vi "WSVCAP SHL Host LL I2C Convert 4 Bytes to Status and Capacitance.vi"(0 "C:1-24 Read Data [U8]":u8[][](array[numeric]) format="%.0x") -> (4 "AD7747 Values":string[][](table))   [LabVIEW 2017]
panel:
  out "Data Headers":u8[](array[numeric])=[1, 2, 3, 4, 5, 6, 7, 8, 9, 10, 11, 12, 12, 14, 15, 16, 17, 18, 19, 20, 21, 22, 23, 24, 25, 26, 27, 28, 29, 30, 31, 32, 33, 34, 35, 36]
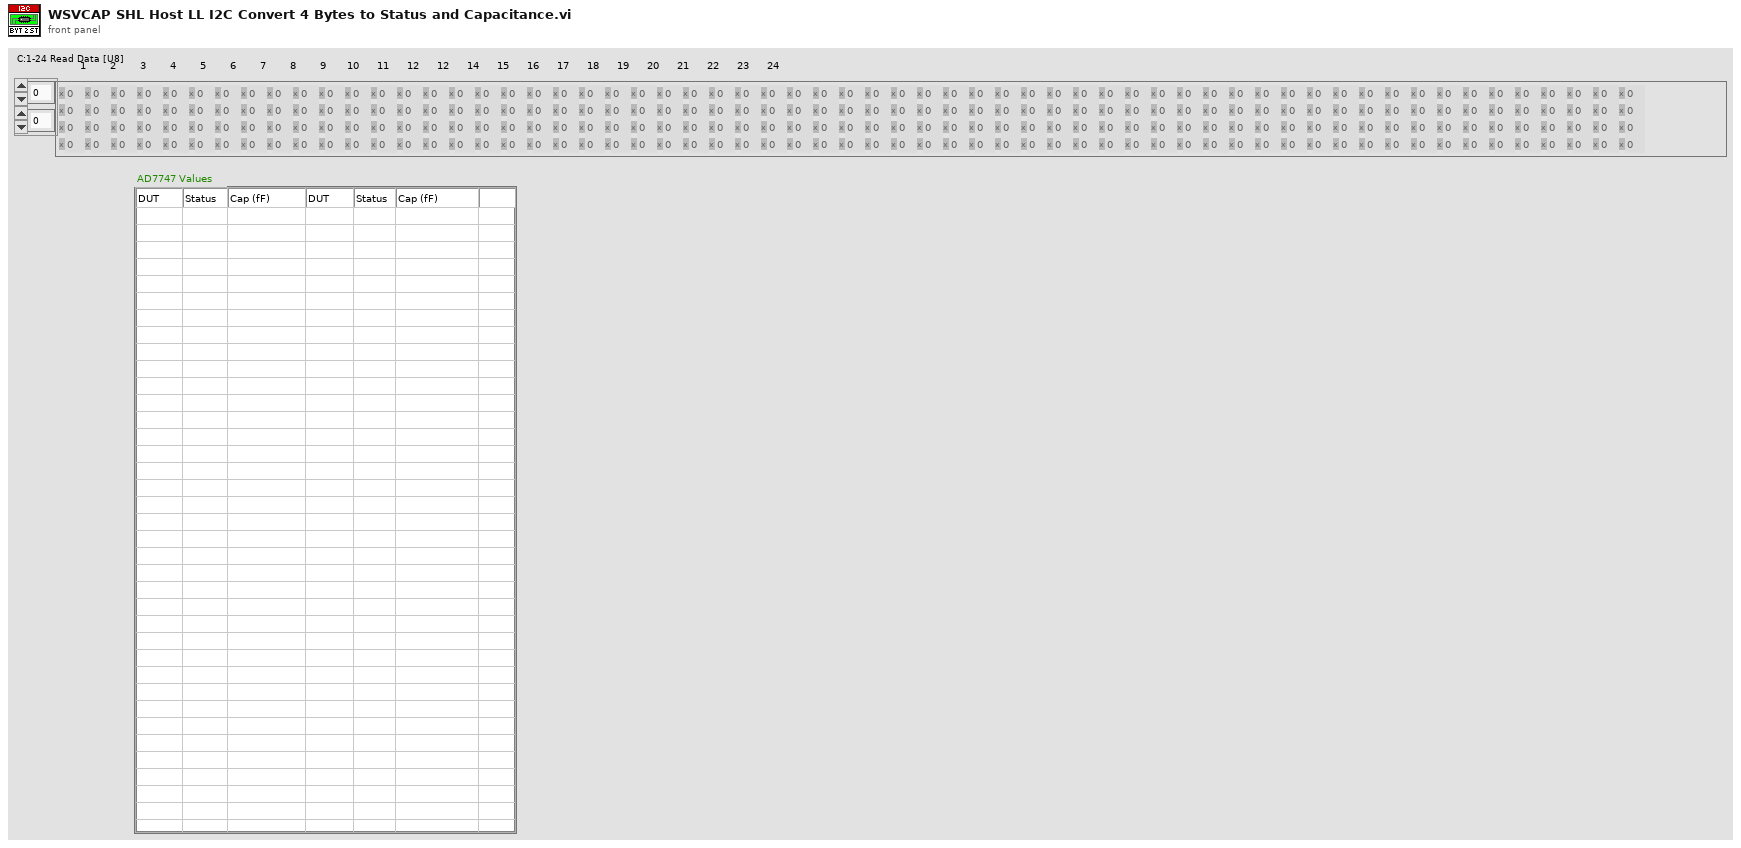
[diagram p1: front panel]
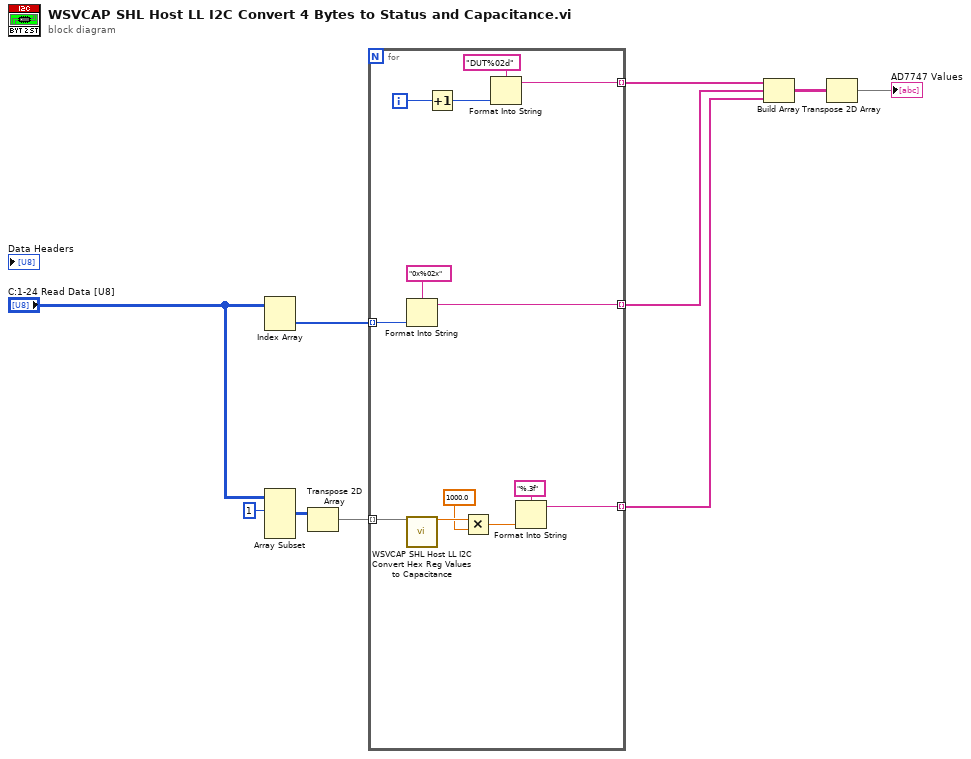
[diagram p0: block diagram]
diagram:
  n1 = Index Array(array="C:1-24 Read Data [U8]") -> (element=w10:u8[])  [unwired: 2 in]
  n2 = Array Subset(array="C:1-24 Read Data [U8]", index (row)=1 ("index")) -> (w8:u8[][])  [unwired: 3 in]
  n3 = Transpose 2D Array(2D array=w8) -> (transposed array=w7:u8[][])
  n4 = for {
    tunnel: w10 -> [w22] mode=indexing
    tunnel: w7 -> [w23] mode=indexing
    tunnel: [w21] -> w3 mode=indexing
    tunnel: [w20] -> w4 mode=indexing
    tunnel: [w15] -> w1 mode=indexing
    i -> [w16]
    n5 = Format Into String(format string="0x%02x", w22) -> (resulting string=w21:string)  [unwired: 2 in, 1 out]
    n6 = call "WSVCAP SHL Host LL I2C Convert Hex Reg Values to Capacitance.vi"("Bytes (H-M-L)"=w23) -> ("Capacitance (pF)"=w13:dbl)  [unwired: 14 in]
    n7 = Increment(x=w16) -> (x+1=w17:i32)
    n8 = Multiply(x=w13, y=1000.0) -> (x*y=w11:dbl)
    n9 = Format Into String(format string="DUT%02d", w17) -> (resulting string=w15:string)  [unwired: 2 in, 1 out]
    n10 = Format Into String(format string="%.3f", w11) -> (resulting string=w20:string)  [unwired: 2 in, 1 out]
  }
  n11 = Build Array(w1, w3, w4) -> (w6:string[][])
  n12 = Transpose 2D Array(2D array=w6) -> (transposed array=→"AD7747 Values":string[][])
